vi "CB Update Controller.vi"(4 "r(k+1)":dbl[](array[numeric]), 6 "Feed Forward":T2, 7 "u_bounds":cluster{"u_max":dbl[], "u_min":dbl[]}, 8 "State Space Model":T1, 9 "x_hat":dbl[](array[numeric]), 10 "r(k)":dbl[](array[numeric]), 11 "K":T2) -> (3 "u":dbl[](array[numeric]))   [LabVIEW 2020]
uses:
  <vilib>/Analysis/Matrix/Datatypes/RealMatrix.ctl
  CB State Space.ctl
  <vilib>/Analysis/baseanly.llb/A x Vector.vi
  <vilib>/Analysis/NI_AALBase.lvlib
  <vilib>/Analysis/Matrix/NI_Matrix.lvlib
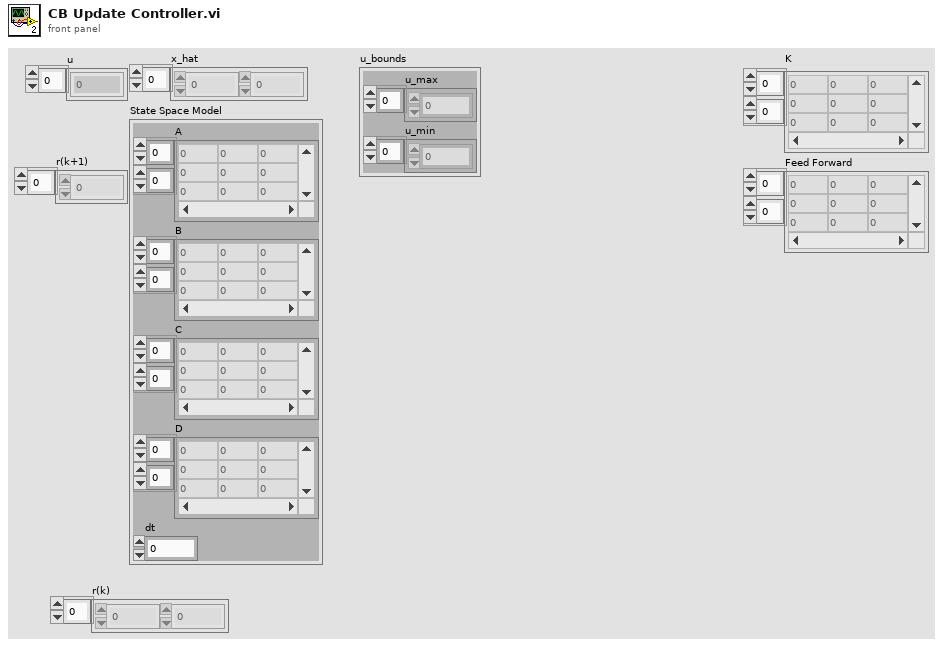
[diagram p1: front panel]
types:
  T1 = typedef "CB State Space.ctl" = cluster{"A":T2, "B":T2, "C":T2, "D":T2, "dt":dbl}
  T2 = typedef "NI_Matrix.lvlib/RealMatrix.ctl" = dbl[][]
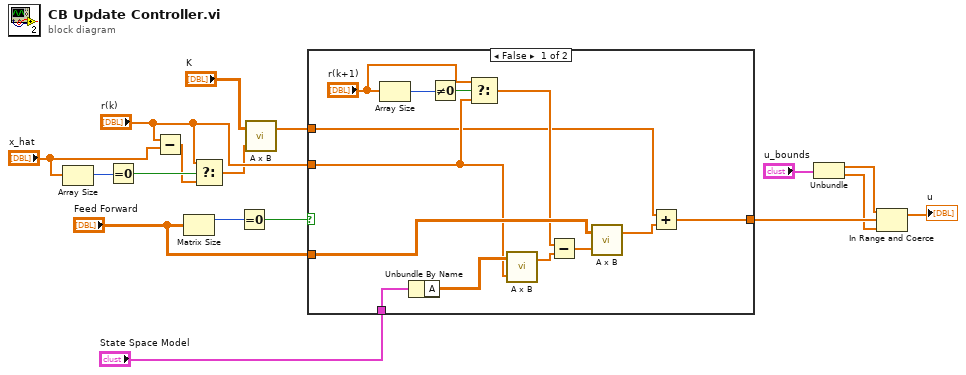
[diagram p0: block diagram]
diagram:
  n1 = Array Size(array="x_hat") -> (size(s)=w10:i32)
  n2 = Equal To 0?(x=w10) -> (x = 0?=w9:bool)
  n3 = Subtract(x="r(k)", y="x_hat") -> (x-y=w7:dbl[])
  n4 = Matrix Size(0:"Feed Forward") -> (1:w16:i32)  [unwired: 1 out]
  n5 = Select(t="r(k)", s=w9, f=w7) -> (s? t:f=w6:dbl[])
  n6 = Equal To 0?(x=w16) -> (x = 0?=w17:bool)
  n7 = call-poly <vilib>:"A x B.vi"("Vector"=w6, "A"="K") -> ("A x Vector"=w12:dbl[])  [unwired: 1 out]
  n8 = case shown="False" w17 {
    tunnel: w12 -> [w18 w31]
    tunnel: "Feed Forward" -> [w26 _]
    tunnel: "State Space Model" -> [w30 _]
    tunnel: "r(k)" -> [w19 _]
    tunnel: [w24 w31] -> w5
    frame False {
      n9 = Array Size(array="r(k+1)") -> (size(s)=w21:i32)
      n10 = Unbundle By Name(w30) -> ("A"=w29:T2)
      n11 = Not Equal To 0?(x=w21) -> (x != 0?=w22:bool)
      n12 = Select(t="r(k+1)", s=w22, f=w19) -> (s? t:f=w20:dbl[])
      n13 = call-poly <vilib>:"A x B.vi"("Vector"=w19, "A"=w29) -> ("A x Vector"=w28:dbl[])  [unwired: 1 out]
      n14 = Subtract(x=w20, y=w28) -> (x-y=w27:dbl[])
      n15 = call-poly <vilib>:"A x B.vi"("Vector"=w27, "A"=w26) -> ("A x Vector"=w25:dbl[])  [unwired: 1 out]
      n16 = Add(x=w18, y=w25) -> (x+y=w24:dbl[])
    }
    frame True {
    }
  }
  n17 = Unbundle("u_bounds") -> ("u_max"=w2:dbl[], "u_min"=w1:dbl[])
  n18 = In Range and Coerce(upper limit=w2, x=w5, lower limit=w1) -> (coerced(x)=→"u":dbl[])  [unwired: 1 out]
